vi "MIDI.vi"(8 "error in (no error)":errorcluster, 11 "Refnum in":refnum<k20>) -> (0 "error out":errorcluster)   [LabVIEW 2014]
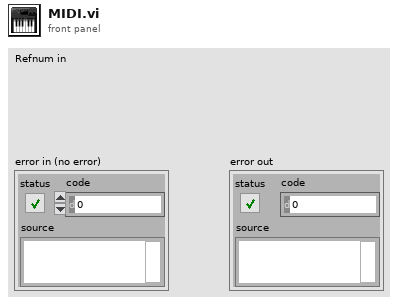
[diagram p1: front panel]
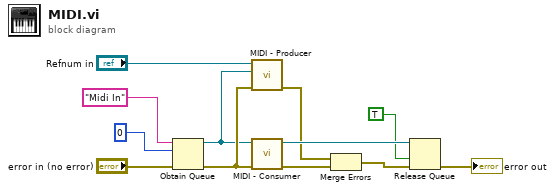
[diagram p0: block diagram]
diagram:
  n1 = Obtain Queue(name (unnamed)="Midi In" ("Queue Name"), element data type=u8 0, error in (no error)="error in (no error)") -> (queue out=w4:refnum<queue>, error out=w10:errorcluster)  [unwired: 2 in, 1 out]
  n2 = call "MIDI - Producer.vi"("error in (no error)"=w10, "queue in"=w4, "Refnum in"="Refnum in") -> ("error out"=w5:errorcluster)  [unwired: 8 in]
  n3 = call "MIDI - Consumer.vi"("error in (no error)"=w10, "Queue in"=w4) -> ("error out"=w7:errorcluster, "Queue out"=w11:refnum<queue>)  [unwired: 8 in]
  n4 = Merge Errors(w5, w7) -> (w6:errorcluster)
  n5 = Release Queue(queue=w11, force destroy? (F)=TRUE, error in (no error)=w6) -> (error out=→"error out":errorcluster)  [unwired: 2 out]
